vi "ReadPartsList_BeforeSelect.vi"(8 "error in":errorcluster, 11 "Default\nJSON Variant in":variant) -> (0 "error out":errorcluster, 3 "Part Names out":string[](array[string]))   [LabVIEW 2015, in "ZenGage v3.0 UI.lvclass"]
uses:
  ZenGage v3.0 UI.lvclass
panel:
  in  "Part Names":string[](array[string])
  in  "?":T1
  out "Variant":variant
  out "VCluster\n out":variant
  out "Error Message":string
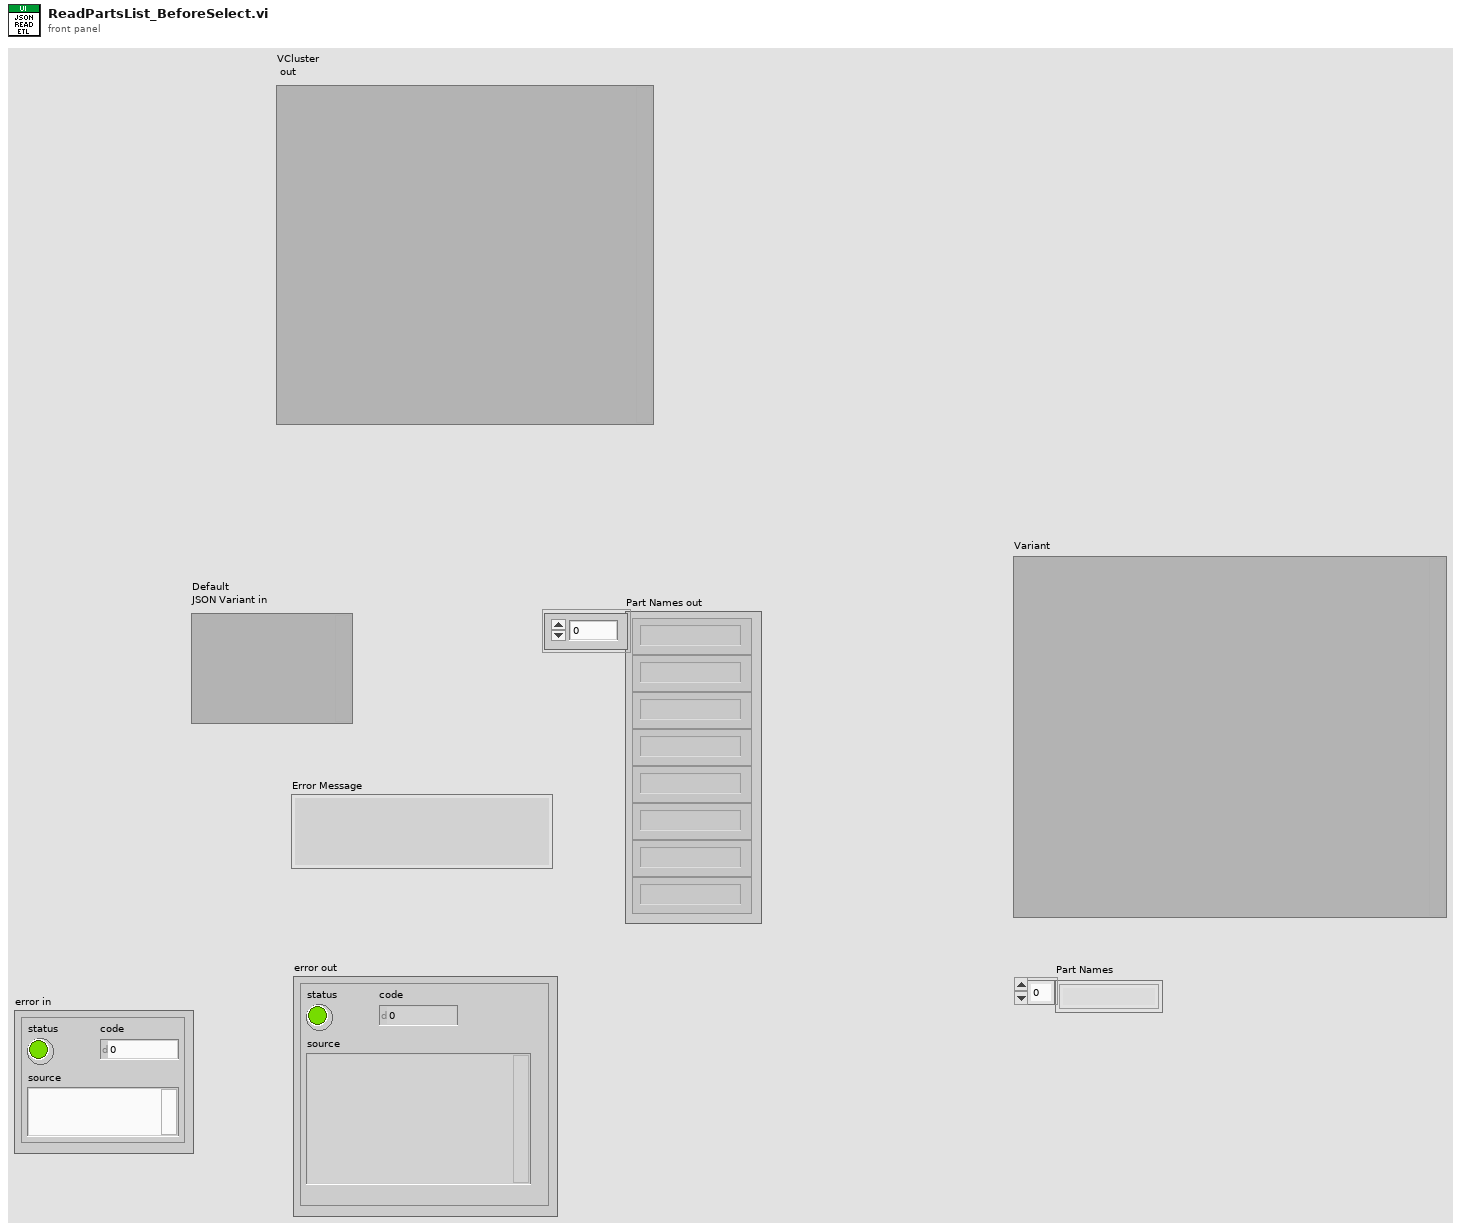
[diagram p1: front panel]
types:
  T1 = cluster{"AlgoParameters":cluster{"PartsList":cluster{"Name":string, "ImageStreams":cluster{"ThreadName":string, "RackEnable":bool, "ThreadId":i32, "RackId":i32, "ImagingViews":cluster{"ViewName":string, "ViewEnable":bool, "ImageID":i32, "CameraID":i32, "CalibrationFilePath":string, "ReferenceCoordSystem":cluster{"Method":cluster{"Algo":string, "BaseReference":cluster{"OriginX":i32, "OriginY":i32, "Angle":dbl, "AxisReference":i32}}, "ROI1":cluster{"ROI":cluster{"Left":i32, "Top":i32, "Right":i32, "Bottom":i32, "Rotation":dbl}, "EdgeOptions":cluster{"EdgePolarity":i32, "KernelSize":i32, "Width":i32, "MinimumEdgeStrength":i32, "InterpolationType":i32, "DataProcessingMethod":i32}, "LineOptions":cluster{"NumberofLines":i32, "Type":i32, "MinScore":i32, "MaxScore":i32, "Orientation":i32, "AngleRange":i32, "AngleTolerance":i32, "StepSize":i32, "MinSNR":i32, "MinPoints":i32, "HoughIterations":i32}, "Process":i32, "StepSize":i32, "SearchDirection":i32, "CircleEdgeOptions":cluster{"SearchDirection":i32, "EdgeOptions":cluster{"EdgePolarity":i32, "KernelSize":i32, "Width":i32, "MinimumEdgeStrength":i32, "InterpolationType":i32, "DataProcessingMethod":i32}}, "CircleFitOptions":cluster{"Process":i32, "StepSize":i32, "MAxPixelRadius":i32}, "CircleSearchDirection":i32, "CurveParameters":cluster{"ExtractionMode":i32, "EdgeThreshold":i32, "EdgeFilterSize":i32, "MinLength":i32, "RowSearchStepSize":i32, "ColSearchStepSize":i32, "MaxEndpointGap":i32, "Closed":bool, "Subpixel":bool}, "MinimumMatchScore":i32, "CircleDescriptor":cluster{"MinRadius":i32, "MaxRadius":i32}, "EllipseDescriptor":cluster{"MinMajorRadius":i32, "MaxMajorRadius":i32, "MinMinorRadius":i32, "MaxMinorRadius":i32}, "ParallelLines":cluster{"First":i32, "Second":i32, "Third":i32}, "OverlayOptions":cluster{"OverlayEnable":bool, "OverlayText":string, "OverlayCoords":i32[], "OverlayAngle":i32, "OverlayTextSize":i32, "OverlayTextColor":string}, "ResultVariableCluster":cluster{"RVName":string, "RVSequence":string, "RVIndex":i32, "RVID":i32, "RVValue":dbl}}, "Name":string}}[]}[], "Measurements":cluster{"RackID":i32, "ImageID":i32, "CameraID":i32, "MeasurementId":i32, "Name":string, "AlgoName":string, "Type":string, "MeasurementEnable":bool, "AlgorithmSequence":cluster{"RefernceEdge":cluster{"Enable":bool, "Method":string, "RefROI":cluster{"Left":i32, "Top":i32, "Right":i32, "Bottom":i32, "Rotation":dbl}, "EdgeOptions":cluster{"EdgePoarity":i32, "KernelSize":i32, "Width":i32, "MinimumEdgeStrength":i32, "InterpolationType":i32, "DataProcessingMethod":i32}, "LineOptions":cluster{"NumberofLines":i32, "Type":i32, "MinScore":i32, "MaxScore":i32, "Orientation":i32, "AngleRange":i32, "AngleTolerance":i32, "StepSize":i32, "MinSNR":i32, "MinPoints":i32, "HoughIterations":i32}, "ResultVariableCluster":cluster{"RVName":string, "RVSequence":string, "RVIndex":i32, "RVID":i32, "RVValue":dbl}, "SearchDirection":i32}, "Measurement":cluster{"ROI1":cluster{"Enable":bool, "ROI":cluster{"Left":i32, "Top":i32, "Right":i32, "Bottom":i32, "Rotation":dbl}, "EdgeOptions":cluster{"EdgePoarity":i32, "KernelSize":i32, "Width":i32, "MinimumEdgeStrength":i32, "InterpolationType":i32, "DataProcessingMethod":i32}, "LineOptions":cluster{"NumberofLines":i32, "Type":i32, "MinScore":i32, "MaxScore":i32, "Orientation":i32, "AngleRange":i32, "AngleTolerance":i32, "StepSize":i32, "MinSNR":i32, "MinPoints":i32, "HoughIterations":i32}, "Process":i32, "StepSize":i32, "SearchDirection":i32, "CircleEdgeOptions":cluster{"SearchDirection":i32, "EdgeOptions":cluster{"EdgePoarity":i32, "KernelSize":i32, "Width":i32, "MinimumEdgeStrength":i32, "InterpolationType":i32, "DataProcessingMethod":i32}}, "CircleFitOptions":cluster{"Process":i32, "StepSize":i32, "MAxPixelRadius":dbl}, "CircleSearchDirection":i32, "CurveParameters":cluster{"ExtractionMode":i32, "EdgeThreshold":i32, "EdgeFilterSize":i32, "MinLength":i32, "RowSearchStepSize":i32, "ColSearchStepSize":i32, "MaxEndpointGap":i32, "Closed":bool, "Subpixel":bool}, "MinimumMatchScore":i32, "CircleDescriptor":cluster{"MinRadius":i32, "MaxRadius":i32}, "EllipseDescriptor":cluster{"MinMajorRadius":i32, "MaxMajorRadius":i32, "MinMinorRadius":i32, "MaxMinorRadius":i32}, "OverlayOptions":cluster{"OverlayEnable":bool, "OverlayText":string, "OverlayCoords":i32[], "OverlayAngle":i32, "OverlayTextSize":i32, "OverlayTextColor":string}, "ResultVariableCluster":cluster{"RVName":string, "RVSequence":string, "RVIndex":i32, "RVID":i32, "RVValue":dbl}}, "ROI2":cluster{"Enable":bool, "ROI":cluster{"Left":i32, "Top":i32, "Right":i32, "Bottom":i32, "Rotation":dbl}, "EdgeOptions":cluster{"EdgePoarity":i32, "KernelSize":i32, "Width":i32, "MinimumEdgeStrength":i32, "InterpolationType":i32, "DataProcessingMethod":i32}, "LineOptions":cluster{"NumberofLines":i32, "Type":i32, "MinScore":i32, "MaxScore":i32, "Orientation":i32, "AngleRange":i32, "AngleTolerance":i32, "StepSize":i32, "MinSNR":i32, "MinPoints":i32, "HoughIterations":i32}, "Process":i32, "StepSize":i32, "SearchDirection":i32, "CircleEdgeOptions":cluster{"SearchDirection":i32, "EdgeOptions":cluster{"EdgePoarity":i32, "KernelSize":i32, "Width":i32, "MinimumEdgeStrength":i32, "InterpolationType":i32, "DataProcessingMethod":i32}}, "CircleFitOptions":cluster{"Process":i32, "StepSize":i32, "MAxPixelRadius":dbl}, "CircleSearchDirection":i32, "CurveParameters":cluster{"ExtractionMode":i32, "EdgeThreshold":i32, "EdgeFilterSize":i32, "MinLength":i32, "RowSearchStepSize":i32, "ColSearchStepSize":i32, "MaxEndpointGap":i32, "Closed":bool, "Subpixel":bool}, "MinimumMatchScore":i32, "CircleDescriptor":cluster{"MinRadius":i32, "MaxRadius":i32}, "EllipseDescriptor":cluster{"MinMajorRadius":i32, "MaxMajorRadius":i32, "MinMinorRadius":i32, "MaxMinorRadius":i32}, "OverlayOptions":cluster{"OverlayEnable":bool, "OverlayText":string, "OverlayCoords":i32[], "OverlayAngle":i32, "OverlayTextSize":i32, "OverlayTextColor":string}, "ResultVariableCluster":cluster{"RVName":string, "RVSequence":string, "RVIndex":i32, "RVID":i32, "RVValue":dbl}}}, "MathExpression":cluster{"Algorithm":string, "MathExpression":string, "ResultVariable":string}}, "CalibrationCoefficients":cluster{"A1":dbl, "A2":dbl, "A3":dbl}, "UserCalibCoefficients":cluster{"UserCorrectionLinearityCoeff":dbl, "UserCorrectionBiasCoeff":dbl}, "SpecValues":cluster{"USL":dbl, "LCL":dbl, "UCL":dbl, "LSL":dbl, "NominalValue":dbl}, "OverlayOptions":cluster{"OverlayEnable":bool, "OverlayText":string, "OverlayCoords":i32[], "OverlayAngle":i32, "OverlayTextSize":i32, "OverlayTextColor":string}, "DatalogEnable":bool, "DisplayIcon":string}[]}[], "AlgoDefaultParameters":cluster{"AlgoName":string, "Enable":bool, "AlgorithmSequenceDefault":cluster{"RefernceEdgeDefault":cluster{"Method":string, "RefROI":cluster{"Left":i32, "Top":i32, "Right":i32, "Bottom":i32, "Rotation":i32}, "EdgeOptions":cluster{"EdgePoarity":i32, "KernelSize":i32, "Width":i32, "MinimumEdgeStrength":i32, "InterpolationType":i32, "DataProcessingMethod":i32}, "LineOptions":cluster{"NumberofLines":i32, "Type":i32, "MinScore":i32, "MaxScore":i32, "Orientation":i32, "AngleRange":i32, "AngleTolerance":i32, "StepSize":i32, "MinSNR":i32, "MinPoints":i32, "HoughIterations":i32}, "SearchDirection":i32}, "MeasurementDefault":cluster{"ROI1":cluster{"ROI":cluster{"Left":i32, "Top":i32, "Right":i32, "Bottom":i32, "Rotation":i32}, "EdgeOptions":cluster{"EdgePoarity":i32, "KernelSize":i32, "Width":i32, "MinimumEdgeStrength":i32, "InterpolationType":i32, "DataProcessingMethod":i32}, "LineOptions":cluster{"NumberofLines":i32, "Type":i32, "MinScore":i32, "MaxScore":i32, "Orientation":i32, "AngleRange":i32, "AngleTolerance":i32, "StepSize":i32, "MinSNR":i32, "MinPoints":i32, "HoughIterations":i32}, "Process":i32, "StepSize":i32, "SearchDirection":i32, "CircleEdgeOptions":cluster{"SearchDirection":i32, "EdgeOptions":cluster{"EdgePoarity":i32, "KernelSize":i32, "Width":i32, "MinimumEdgeStrength":i32, "InterpolationType":i32, "DataProcessingMethod":i32}}, "CircleFitOptions":cluster{"Process":i32, "StepSize":i32, "MAxPixelRadius":i32}, "CircleSearchDirection":i32, "CurveParameters":cluster{"ExtractionMode":i32, "EdgeThreshold":i32, "EdgeFilterSize":i32, "MinLength":i32, "RowSearchStepSize":i32, "ColSearchStepSize":i32, "MaxEndpointGap":i32, "Closed":i32, "Subpixel":i32}, "MinimumMatchScore":i32, "CircleDescriptor":cluster{"MinRadius":i32, "MaxRadius":i32}, "EllipseDescriptor":cluster{"MinMajorRadius":i32, "MaxMajorRadius":i32, "MinMinorRadius":i32, "MaxMinorRadius":i32}, "OverlayOptions":cluster{"OverlayEnable":bool, "OverlayText":string, "OverlayCoords":i32[], "OverlayAngle":i32, "OverlayTextSize":i32, "OverlayTextColor":string}, "ResultVariable":string}, "ROI2":cluster{"ROI":cluster{"Left":i32, "Top":i32, "Right":i32, "Bottom":i32, "Rotation":i32}, "EdgeOptions":cluster{"EdgePoarity":i32, "KernelSize":i32, "Width":i32, "MinimumEdgeStrength":i32, "InterpolationType":i32, "DataProcessingMethod":i32}, "LineOptions":cluster{"NumberofLines":i32, "Type":i32, "MinScore":i32, "MaxScore":i32, "Orientation":i32, "AngleRange":i32, "AngleTolerance":i32, "StepSize":i32, "MinSNR":i32, "MinPoints":i32, "HoughIterations":i32}, "Process":i32, "StepSize":i32, "SearchDirection":i32, "CircleEdgeOptions":cluster{"SearchDirection":i32, "EdgeOptions":cluster{"EdgePoarity":i32, "KernelSize":i32, "Width":i32, "MinimumEdgeStrength":i32, "InterpolationType":i32, "DataProcessingMethod":i32}}, "CircleFitOptions":cluster{"Process":i32, "StepSize":i32, "MaxPixelRadius":i32}, "CircleSearchDirection":i32, "CurveParameters":cluster{"ExtractionMode":i32, "EdgeThreshold":i32, "EdgeFilterSize":i32, "MinLength":i32, "RowSearchStepSize":i32, "ColSearchStepSize":i32, "MaxEndpointGap":i32, "Closed":i32, "Subpixel":i32}, "MinimumMatchScore":i32, "CircleDescriptor":cluster{"MinRadius":i32, "MaxRadius":i32}, "EllipseDescriptor":cluster{"MinMajorRadius":i32, "MaxMajorRadius":i32, "MinMinorRadius":i32, "MaxMinorRadius":i32}, "OverlayOptions":cluster{"OverlayEnable":bool, "OverlayText":string, "OverlayCoords":i32[], "OverlayAngle":i32, "OverlayTextSize":i32, "OverlayTextColor":string}, "ResultVariable":string}}, "MathExpressionDefault":cluster{"Algorithm":string, "MathExpression":string, "ResultVariable":string}}, "CalibrationCoefficients":cluster{"A1":i32, "A2":dbl, "A3":dbl}, "UserCalibCoefficients":cluster{"UserCorrectionBiasCoeff":i32, "UserCorrectionLinearityCoeff":i32}, "ControlLimitsViolationThreshold":cluster{"LCL":i32, "UCL":i32}, "SpecificationLimitViolationThreshold":cluster{"LSL":i32, "USL":i32}, "OverlayOptions":cluster{"OverlayEnable":bool, "OverlayText":string, "OverlayCoords":i32[], "OverlayAngle":i32, "OverlayTextSize":i32, "OverlayTextColor":string}, "DatalogEnable":bool, "DisplayIcon":string}}}
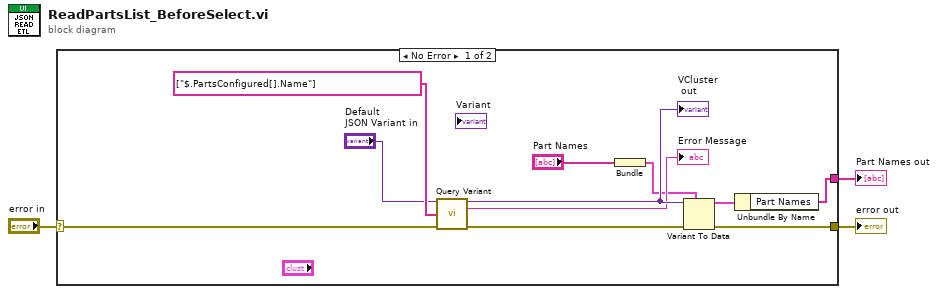
[diagram p0: block diagram]
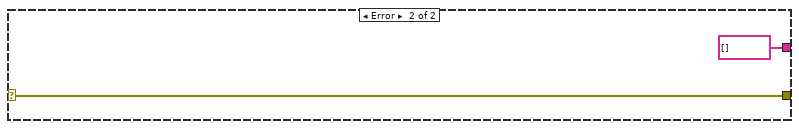
[diagram p2: hidden frame]
diagram:
  n1 = case shown="No Error" "error in" {
    selector: "error in" -> [w10 w16]
    tunnel: [w12 w16] -> w3
    tunnel: [w5 string[] [] ("Part Names")] -> w1
    frame No Error {
      n2 = call <vilib>:"Query Variant.vi"("VCluster in"="Default\nJSON Variant in", "pathList"=string[] ["$.PartsConfigured[].Name"], "error IO"=w10) -> ("VCluster\n out"=w14:variant, "Error Message"=→"Error Message":string, "error out"=w13:errorcluster)  [unwired: 9 in, 1 out]
      "VCluster\n out" <- w14
      n3 = Bundle("Part Names"="Part Names") -> (w7:cluster{"Part Names":string[]})  [unwired: 1 in]
      n4 = Variant To Data(error in=w13, type=w7, Variant=w14) -> (data=w6:cluster{"Part Names":string[]}, error out=w12:errorcluster)
      n5 = Unbundle By Name(w6) -> ("Part Names"=w5:string[])
    }
    frame Error {
    }
  }
  "error out" <- w3
  "Part Names out" <- w1
